vi "Read Safe Mode.vi"(8 "error in (no error)":errorcluster, 11 "Ancestor in":refnum<class "Ancestor.lvclass">) -> (0 "error out":errorcluster, 2 "Safe Mode":bool, 3 "Ancestor out":refnum<class "Ancestor.lvclass">)   [LabVIEW 2026, in "TALOS.lvlib" / "Ancestor.lvlib" / "Ancestor.lvclass"]
uses:
  Ancestor.lvclass
  Ancestor.lvclass/Ancestor.ctl
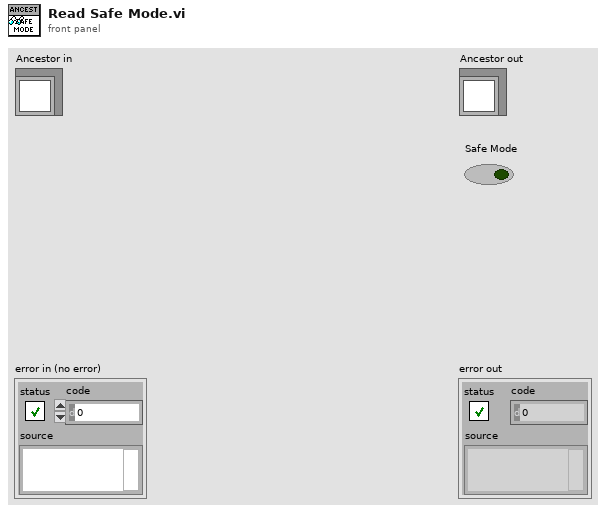
[diagram p1: front panel]
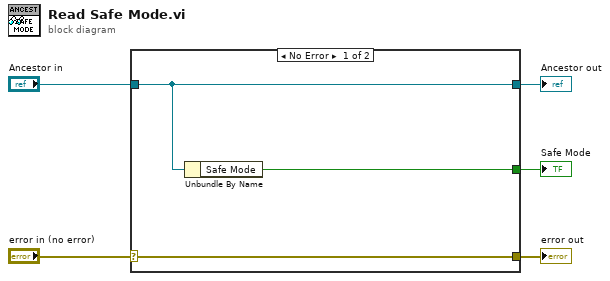
[diagram p0: block diagram]
diagram:
  n1 = case shown="No Error" "error in (no error)" {
    selector: "error in (no error)" -> [w8 w9]
    tunnel: [w8 w9] -> w4
    tunnel: [w7 w10] -> w2
    tunnel: "Ancestor in" -> [w7 w10]
    tunnel: [w6 _] -> w1
    frame No Error {
      n2 = Unbundle By Name(w7) -> ("Safe Mode"=w6:bool)
    }
    frame Error {
    }
  }
  "error out" <- w4
  "Ancestor out" <- w2
  "Safe Mode" <- w1
